vi "HV_ISet_Multi.vi"(8 "Currents":string[](array[string])=["200", "200", "200", "200", "200", "200", "200", "200", "200", "200", "200", "200"], 11 "Channels":string[](array[string])=["0", "1", "2", "3", "4", "5", "6", "7", "8", "9", "10", "11"]) -> (3 "Outputs":string[](array[string]))   [LabVIEW 2019]
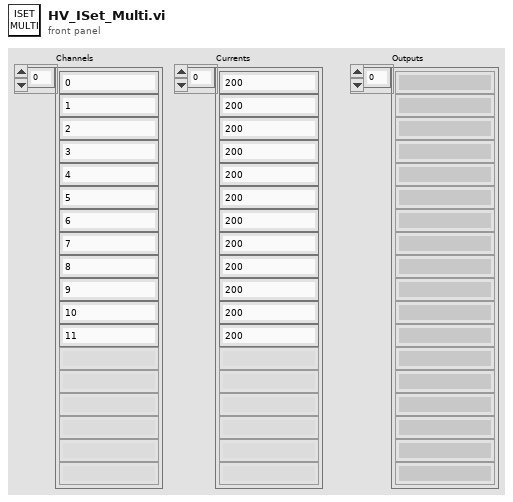
[diagram p1: front panel]
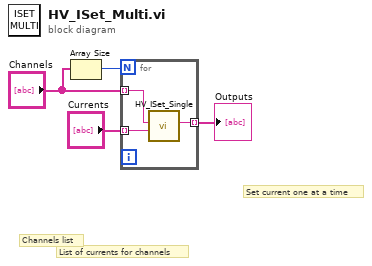
[diagram p0: block diagram]
diagram:
  # "Set current one at a time"
  # "List of currents for channels"
  # "Channels list"
  n1 = Array Size(array="Channels") -> (size(s)=w4:i32)
  n2 = for {
    N: w4 -> [_]
    tunnel: "Channels" -> [w7] mode=indexing
    tunnel: [w6] -> w2 mode=indexing
    tunnel: "Currents" -> [w5] mode=indexing
    n3 = call "HV_ISet_Single.vi"("Current"=w5, "Channel"=w7) -> ("Output"=w6:string)  [unwired: 9 in]
  }
  "Outputs" <- w2
